vi "Configure Frequency Sweep.vi"(4 "Stop  Frequency  (1000.0 Hz)":dbl=1000.0 format="%#.6g", 6 "Start Frequency (100.0 Hz)":dbl=100.0 format="%#.6g", 7 "Enable Frequency Sweep (T:Enable)":bool=TRUE, 8 "error in (no error)":errorcluster, 9 "Sweep Time (1.00 s)":dbl=1.0 min=0.001 max=500.0 format="%#.6g", 10 "Sweep Spacing (0: Linear)":enum16{"Linear", "Log"}(ring), 11 "VISA resource name":refnum<visa-resource-name>) -> (0 "error out":errorcluster, 3 "VISA resource name out":refnum<visa-resource-name>)   [LabVIEW 2017, in "Keithley 3390.lvlib"]
doc: "Configures and enables a frequency sweep. In the frequency sweep mode, the function generator steps from the start frequency to the stop frequency at a sweep rate."
uses:
  Keithley 3390.lvlib
panel:
  in  "Marker Frequency (550 Hz)":dbl=550.0
  in  "Enable Marker Frequency (T:Enable)":bool
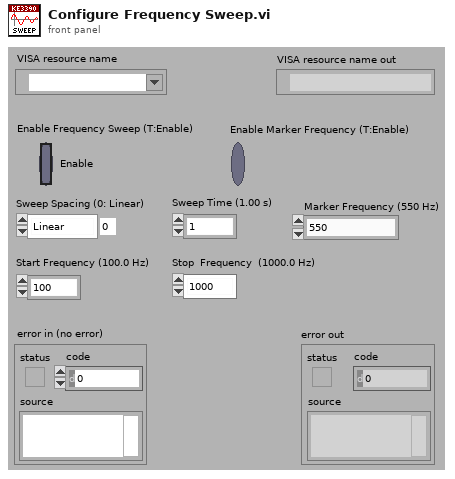
[diagram p1: front panel]
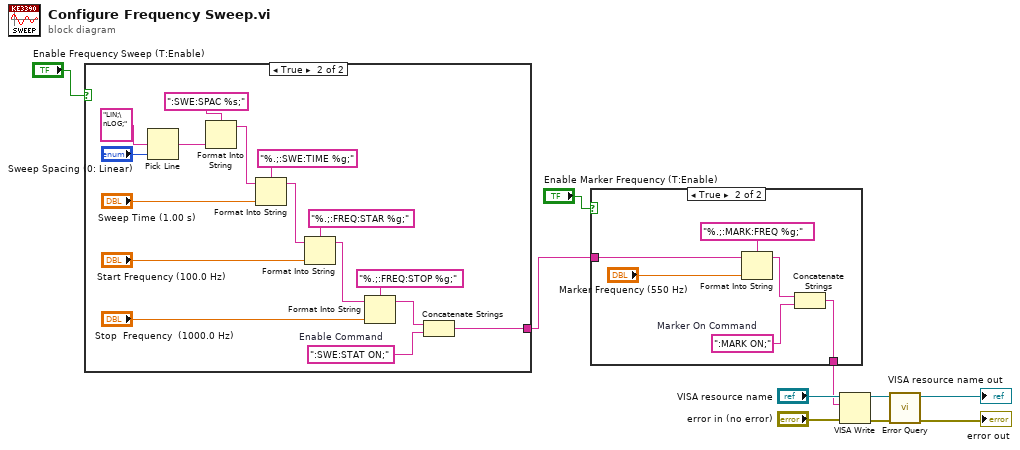
[diagram p0: block diagram]
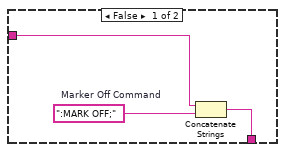
[diagram p2: hidden frame]
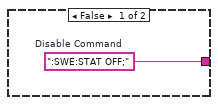
[diagram p3: hidden frame]
diagram:
  n1 = case shown="True" "Enable Frequency Sweep (T:Enable)" {
    tunnel: [w11 w14] -> w2
    frame False {
      w11 = ":SWE:STAT OFF;"  # Disable Command
    }
    frame True {
      w12 = ":SWE:STAT ON;"  # Enable Command
      n2 = Pick Line(multi-line string="LIN;\nLOG;", line index="Sweep Spacing (0: Linear)") -> (output string=w18:string)  [unwired: 1 in]
      n3 = Format Into String(format string=":SWE:SPAC %s;", w18) -> (resulting string=w17:string)  [unwired: 2 in, 1 out]
      n4 = Format Into String(format string="%.;:SWE:TIME %g;", initial string=w17, "Sweep Time (1.00 s)") -> (resulting string=w24:string)  [unwired: 1 in, 1 out]
      n5 = Format Into String(format string="%.;:FREQ:STAR %g;", initial string=w24, "Start Frequency (100.0 Hz)") -> (resulting string=w21:string)  [unwired: 1 in, 1 out]
      n6 = Format Into String(format string="%.;:FREQ:STOP %g;", initial string=w21, "Stop  Frequency  (1000.0 Hz)") -> (resulting string=w13:string)  [unwired: 1 in, 1 out]
      n7 = Concatenate Strings(w13, w12) -> (w14:string)
    }
  }
  n8 = case shown="True" "Enable Marker Frequency (T:Enable)" {
    tunnel: w2 -> [w29 w32]
    tunnel: [w30 w31] -> w1
    frame False {
      w28 = ":MARK OFF;"  # Marker Off Command
      n9 = Concatenate Strings(w29, w28) -> (w30:string)
    }
    frame True {
      w33 = ":MARK ON;"  # Marker On Command
      n10 = Format Into String(format string="%.;:MARK:FREQ %g;", initial string=w32, "Marker Frequency (550 Hz)") -> (resulting string=w34:string)  [unwired: 1 in, 1 out]
      n11 = Concatenate Strings(w34, w33) -> (w31:string)
    }
  }
  n12 = VISA Write(VISA resource name="VISA resource name", write buffer=w1, error in (no error)="error in (no error)") -> (VISA resource name out=w8:refnum<visa-resource-name>, error out=w6:errorcluster)  [unwired: 1 out]
  n13 = call "Error Query.vi"("error in (no error)"=w6, "VISA resource name"=w8) -> ("error out"=→"error out":errorcluster, "VISA resource name out"=→"VISA resource name out":refnum<visa-resource-name>)  [unwired: 6 in, 2 out]
